vi "thcd_400_main.vi"(3 "variable_ref":T1) -> ()   [LabVIEW 2019]
uses:
  thcd_controls/ctrl_chn_thcd.ctl
  thcd_controls/variable_reference.ctl
  thcd_controls/ctrl_sms_thcd.ctl
  thcd_commands/thcd_set_samp.vi
panel:
  out "thcd_st_ch2":bool caption="Status"
  out "thcd_res_msg_ch2":string caption="Msg"
  in  "thcd_val_ch2":dbl caption="SP (V)" min=0.0 max=100.0 step=1.0 format="%#.6g"
  in  "set_ch2":bool
  out "Last Updated":timestamp format="%<%Y-%m-%d %H:%M:%S>T"
  out "Sensor data":cluster{cluster{"X":dbl, "Y":dbl}[]}[](graph)
  out "thcd_st":bool caption="Status"
  out "thcd_res_msg":string caption="Msg"
  in  "thcd_val":dbl caption="SP (V)" min=0.0 max=100.0 step=1.0 format="%#.6g"
  in  "milliseconds to wait":u32=1000
  out "thcd_res_4":T3
  out "thcd_res_3":T3
  out "thcd_res_2":T3
  out "thcd_res_1":T3
  in  "getstat":bool
  in  "set":bool
  in  "read":bool
  out "res_ch3":dbl
  out "res_ch2":dbl
  out "res_ch1":dbl
  in  "Baud_rate":u32(ring)=9600 items=["9.6KHz"=9600, "19.2KHz"=19200]
  in  "thcd_visa":refnum<visa-resource-name>="COM13"
  in  "Init Devices":bool
  in  "Exit":bool
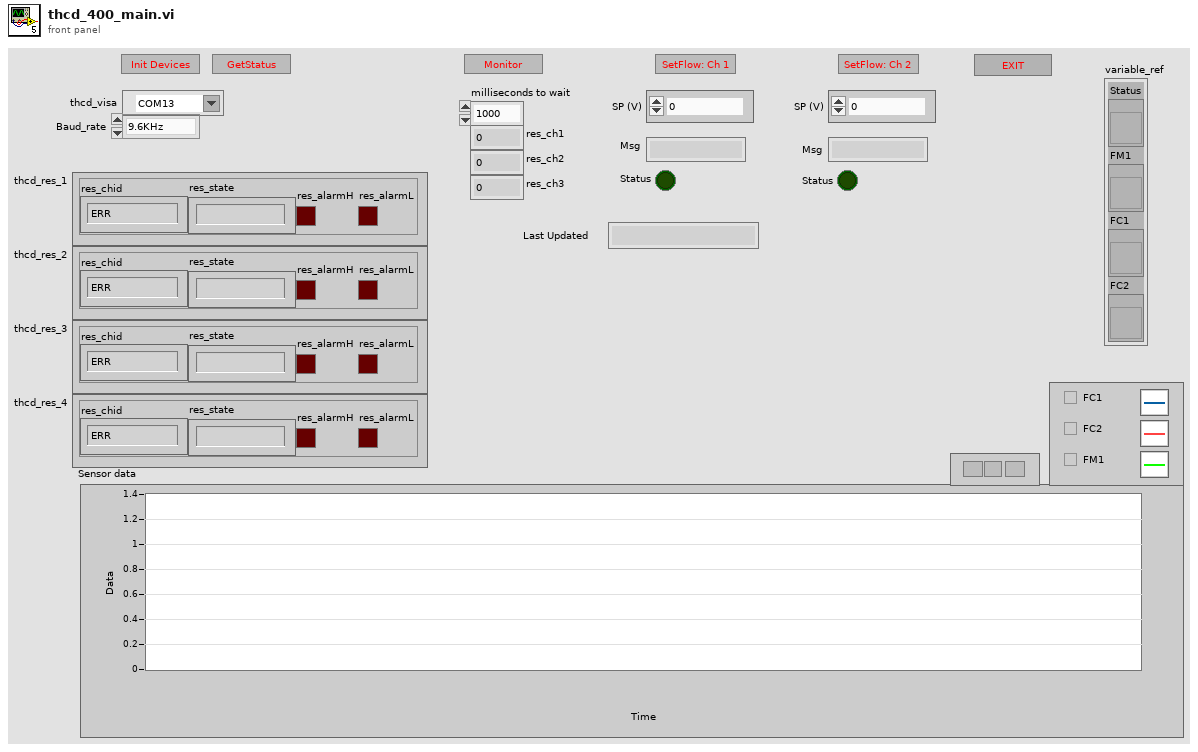
[diagram p1: front panel]
types:
  T1 = typedef "variable_reference.ctl" = cluster{"Status":refnum<vi>, "FM1":refnum<vi>, "FC1":refnum<vi>, "FC2":refnum<vi>}
  T2 = typedef "ctrl_chn_thcd.ctl" = enum8{"ERR", "1", "2", "3", "4"}
  T3 = cluster{"res_chid":T2, "res_state":string, "res_alarmH":bool, "res_alarmL":bool}
  T4 = typedef "ctrl_sms_thcd.ctl" = enum16{"idle", "init", "exit", "read", "set", "set_ch2", "getstat"}
  T5 = enum16{"SetPoint", "AlarmH", "AlarmL", "Multiplier", "CalibValue"}
  T6 = cluster{"res_chid":T2, "res_val":dbl, "res_uom":string, "res_gid":string}[]
  T7 = cluster{"res_chid":T2, "res_val":dbl, "res_uom":string, "res_gid":string}
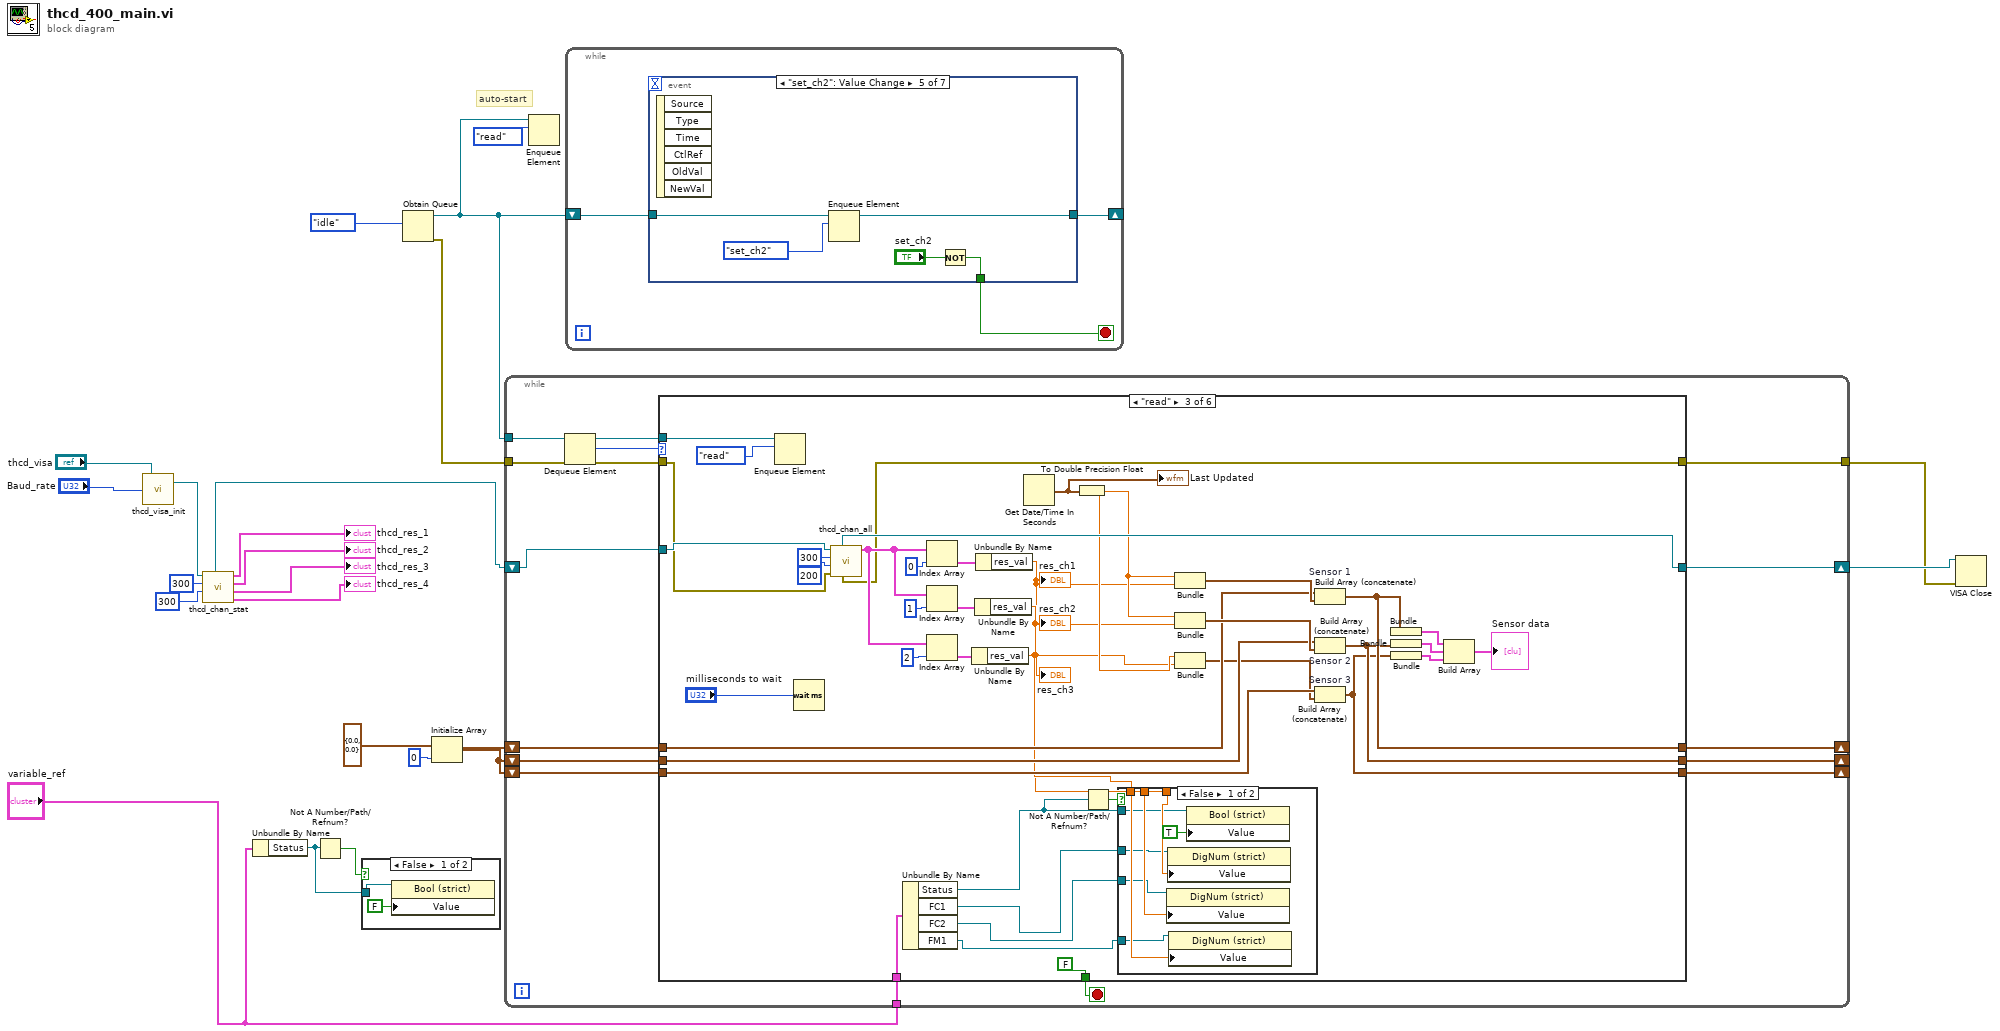
[diagram p0: block diagram]
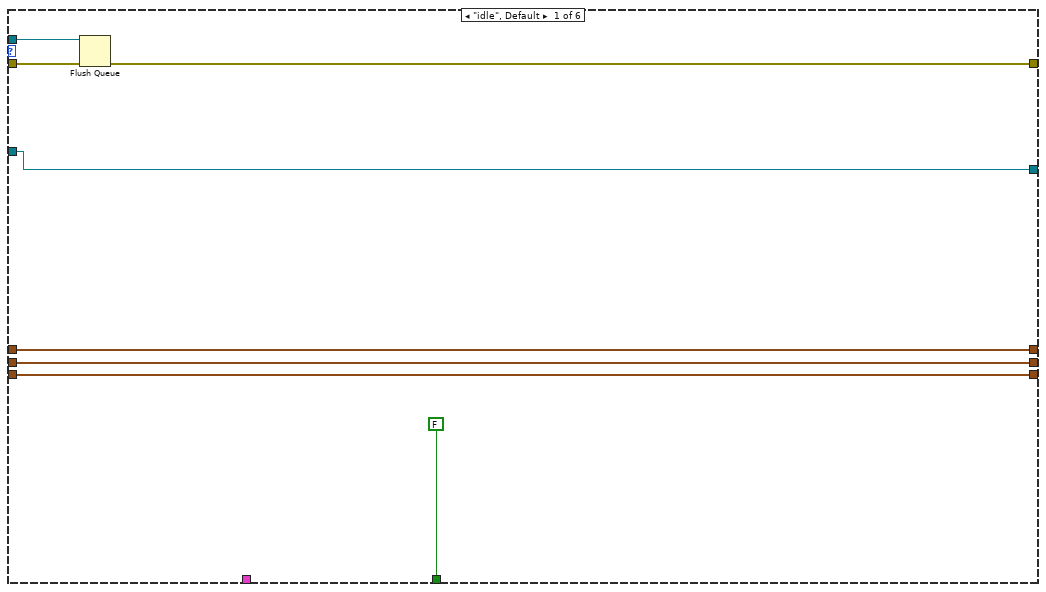
[diagram p3: hidden frame]
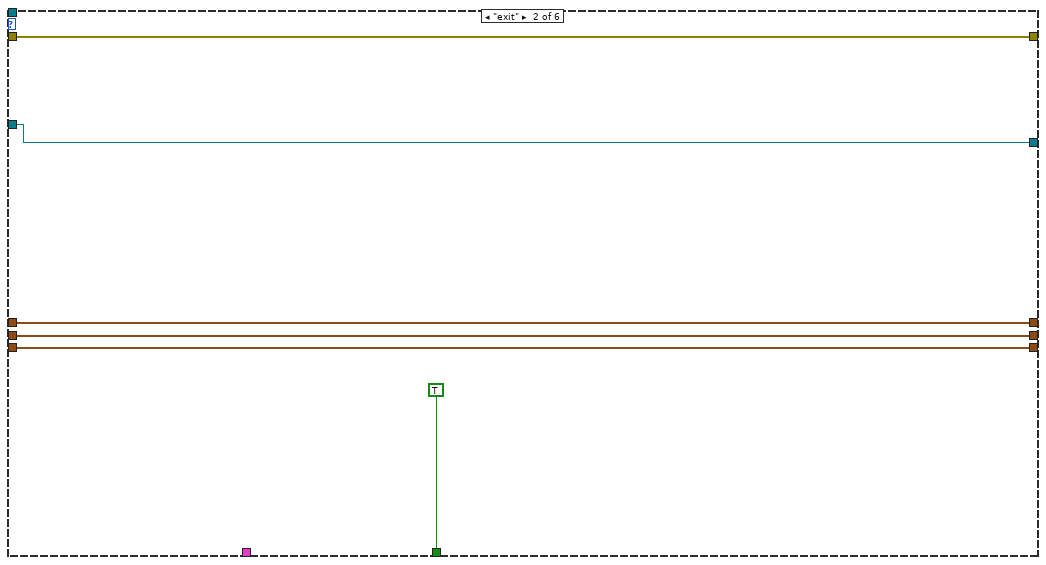
[diagram p4: hidden frame]
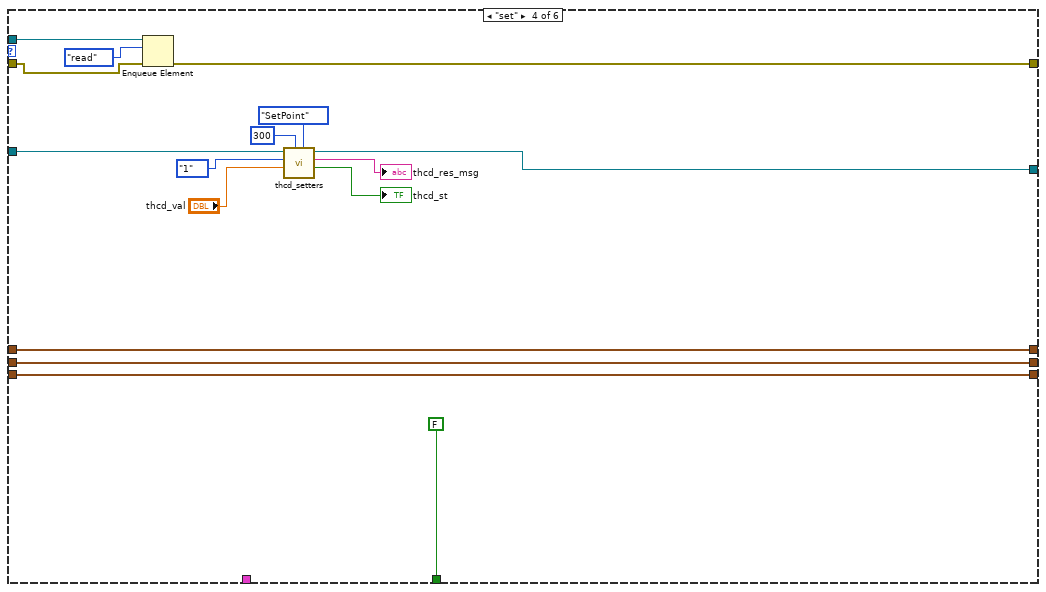
[diagram p6: hidden frame]
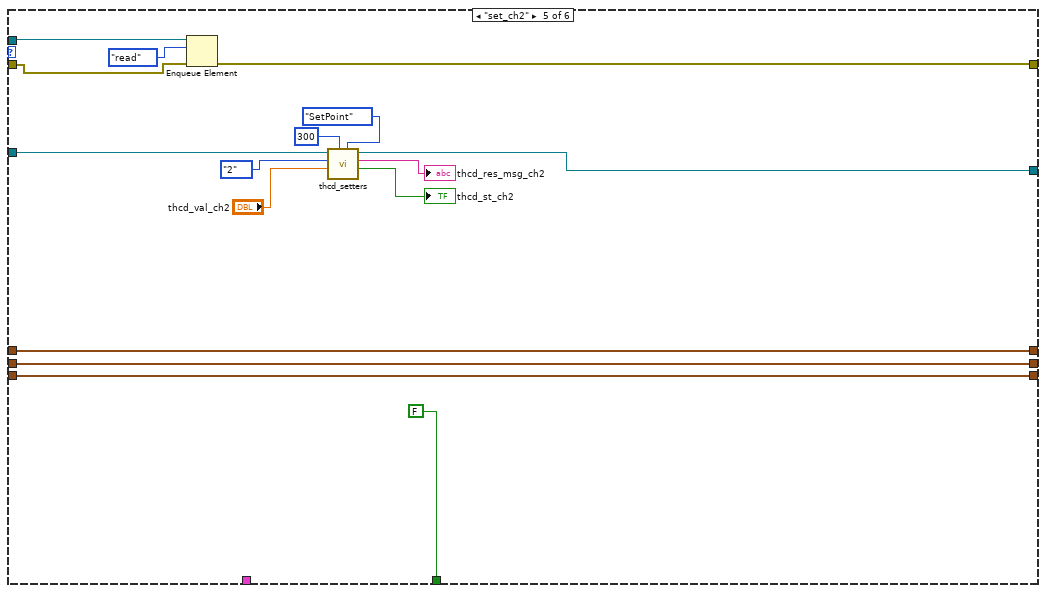
[diagram p7: hidden frame]
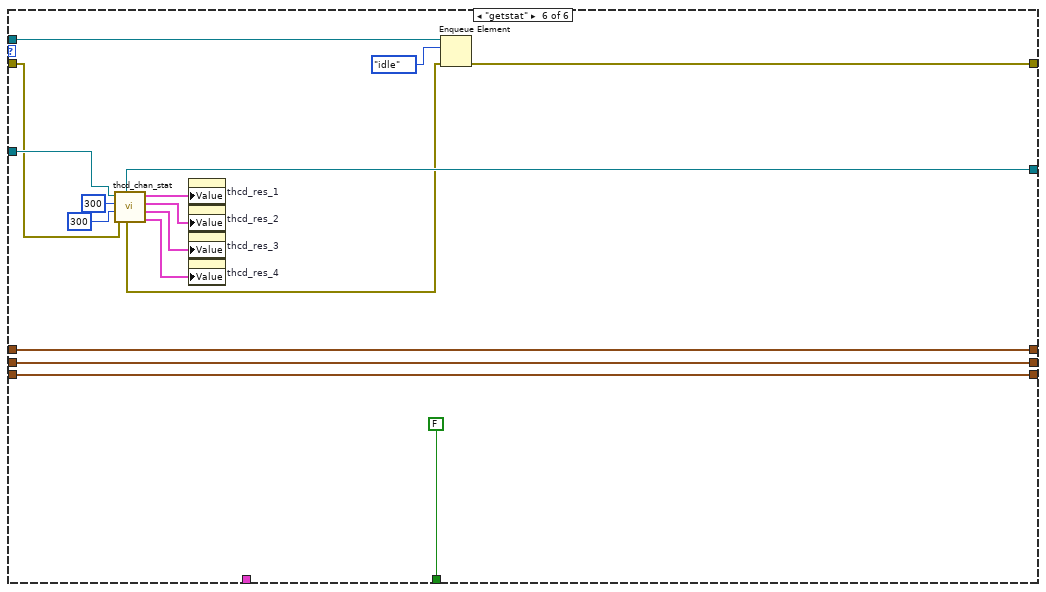
[diagram p8: hidden frame]
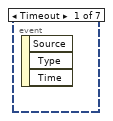
[diagram p9: hidden frame]
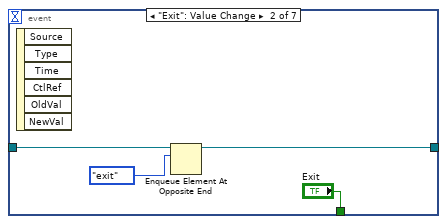
[diagram p10: hidden frame]
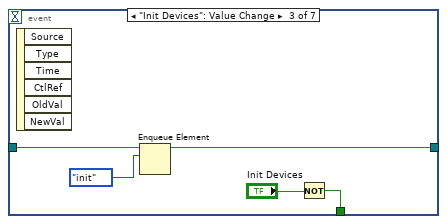
[diagram p11: hidden frame]
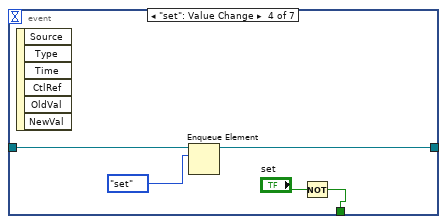
[diagram p12: hidden frame]
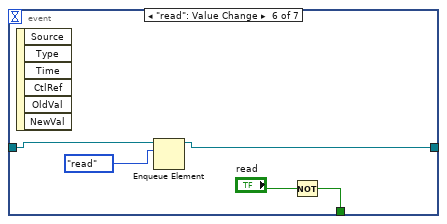
[diagram p13: hidden frame]
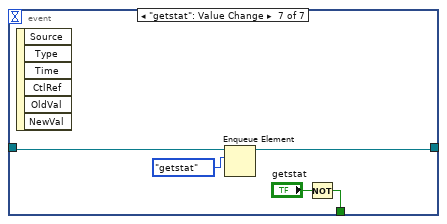
[diagram p14: hidden frame]
diagram:
  # "auto-start"
  n1 = call "thcd_visa_init.vi"("Serial Settings:Baud Rate"="Baud_rate", "thcd_visa"="thcd_visa") -> ("thcd_visa"=w9:refnum<visa-resource-name>)  [unwired: 1 in, 1 out]
  n2 = call "thcd_chan_stat.vi"("thcd_b2r"=u32 300, "thcd_delay"=u32 300, "thcd_visa"=w9) -> ("thcd_res_4"=→"thcd_res_4":T3, "thcd_res_3"=→"thcd_res_3":T3, "thcd_res_2"=→"thcd_res_2":T3, "thcd_res_1"=→"thcd_res_1":T3, "thcd_visa"=w8:refnum<visa-resource-name>)  [unwired: 1 in, 3 out]
  n3 = Unbundle By Name("variable_ref") -> ("Status"=w2:refnum<vi>)
  n4 = Not A Number/Path/Refnum?(number/path/refnum=w2) -> (NaN/Path/Refnum?=w1:bool)
  n5 = case shown="False" w1 {
    tunnel: w2 -> [w24 _]
    frame False {
      n6 = property class="Bool (strict)"(reference=w24, "Value"=FALSE) -> ()  [unwired: 1 in, 2 out]
    }
    frame True {
    }
  }
  n7 = Obtain Queue(element data type=ctrl_sms_thcd."idle" ("Enum")) -> (queue out=w6:refnum<queue>, error out=w21:errorcluster)  [unwired: 4 in, 1 out]
  n8 = Initialize Array(cluster{"X":dbl, "Y":dbl} {"X"=0.0, "Y"=0.0}, 0 ("dimension size")) -> (w18:cluster{"X":dbl, "Y":dbl}[])
  n9 = while {
    tunnel: w21 -> [w38]
    tunnel: [w35] -> w3
    tunnel: w6 -> [w39]
    shift-right: [w26] -> w4
    shift-left: w8 -> [w33]
    shift-right: [w29] -> _
    shift-left: w18 -> [w32]
    shift-right: [w28] -> _
    shift-left: w18 -> [w31]
    shift-right: [w27] -> _
    shift-left: w18 -> [w30]
    tunnel: "variable_ref" -> [w25]
    stop <- w40 stop-if-true
    n10 = Dequeue Element(queue=w39, error in (no error)=w38) -> (queue out=w34:refnum<queue>, element=w37:T4, error out=w36:errorcluster)  [unwired: 1 in, 1 out]
    n11 = case shown="\"read\"" w37 {
      tunnel: w34 -> [w47 _ w79 w117 w128 w151]
      tunnel: [FALSE TRUE FALSE FALSE FALSE FALSE] -> w40
      tunnel: w36 -> [w46 w53 w94 w116 w127 w137]
      tunnel: [w45 w53 w83 w115 w126 w150] -> w35
      tunnel: [w44 w52 w91 w113 w120 w142] -> w26
      tunnel: w33 -> [w44 w52 w95 w114 w125 w143]
      tunnel: w32 -> [w43 w51 w72 w106 w123 w148]
      tunnel: w31 -> [w42 w50 w71 w105 w122 w147]
      tunnel: w30 -> [w41 w49 w70 w104 w121 w146]
      tunnel: [w43 w51 w67 w106 w123 w148] -> w29
      tunnel: [w42 w50 w66 w105 w122 w147] -> w28
      tunnel: [w41 w49 w65 w104 w121 w146] -> w27
      tunnel: w25 -> [_ _ w59 _ _ _]
      frame "idle", Default {
        n12 = Flush Queue(queue=w47, error in (no error)=w46) -> (error out=w45:errorcluster)  [unwired: 2 out]
      }
      frame "exit" {
      }
      frame "read" {
        n13 = Enqueue Element(queue=w79, element=ctrl_sms_thcd."read") -> ()  [unwired: 2 in, 3 out]
        n14 = Wait (ms)(milliseconds to wait="milliseconds to wait") -> ()  [unwired: 1 out]
        n15 = call "thcd_chan_all.vi"("err_in"=w94, "thcd_b2r"=u32 200, "thcd_delay"=u32 300, "thcd_visa"=w95) -> ("thcd_res"=w84:T6, "err_out"=w83:errorcluster, "thcd_visa"=w91:refnum<visa-resource-name>)  [unwired: 3 in, 2 out]
        n16 = Unbundle By Name(w59) -> ("Status"=w60:refnum<vi>, "FC1"=w61:refnum<vi>, "FC2"=w62:refnum<vi>, "FM1"=w63:refnum<vi>)
        n17 = Index Array(array=w84, index=0) -> (element=w89:T7)
        n18 = Index Array(array=w84, index=1) -> (element=w88:T7)
        n19 = Index Array(array=w84, index=2) -> (element=w87:T7)
        n20 = Unbundle By Name(w87) -> ("res_val"=w58:dbl)
        "res_ch3" <- w58
        n21 = Unbundle By Name(w88) -> ("res_val"=w57:dbl)
        "res_ch2" <- w57
        n22 = Unbundle By Name(w89) -> ("res_val"=w56:dbl)
        "res_ch1" <- w56
        n23 = Get Date/Time In Seconds() -> (seconds since 1Jan1904=w55:timestamp)
        "Last Updated" <- w55
        n24 = To Double Precision Float(number=w55) -> (double precision float=w73:dbl)
        n25 = Not A Number/Path/Refnum?(number/path/refnum=w60) -> (NaN/Path/Refnum?=w64:bool)
        n26 = case shown="False" w64 {
          tunnel: w56 -> [w103 _]
          tunnel: w57 -> [w102 _]
          tunnel: w58 -> [w101 _]
          tunnel: w61 -> [w100 _]
          tunnel: w62 -> [w99 _]
          tunnel: w63 -> [w98 _]
          tunnel: w60 -> [w97 _]
          frame False {
            n27 = property class="DigNum (strict)"(reference=w99, "Value"=w102) -> ()  [unwired: 1 in, 2 out]
            n28 = property class="DigNum (strict)"(reference=w100, "Value"=w103) -> ()  [unwired: 1 in, 2 out]
            n29 = property class="DigNum (strict)"(reference=w98, "Value"=w101) -> ()  [unwired: 1 in, 2 out]
            n30 = property class="Bool (strict)"(reference=w97, "Value"=TRUE) -> ()  [unwired: 1 in, 2 out]
          }
          frame True {
          }
        }
        n31 = Bundle(w73, "res_val"=w56) -> (w78:cluster{dbl, "res_val":dbl})  [unwired: 1 in]
        n32 = Bundle(w73, "res_val"=w57) -> (w74:cluster{dbl, "res_val":dbl})  [unwired: 1 in]
        n33 = Bundle(w73, "res_val"=w58) -> (w69:cluster{dbl, "res_val":dbl})  [unwired: 1 in]
        n34 = Build Array (concatenate) "Sensor 1"(w72, w78) -> (w67:cluster{"X":dbl, "res_val":dbl}[])
        n35 = Build Array (concatenate) "Sensor 2"(w71, w74) -> (w66:cluster{"X":dbl, "res_val":dbl}[])
        n36 = Build Array (concatenate) "Sensor 3"(w70, w69) -> (w65:cluster{"X":dbl, "res_val":dbl}[])
        n37 = Bundle(w67) -> (w77:cluster{cluster{"X":dbl, "res_val":dbl}[]})  [unwired: 1 in]
        n38 = Bundle(w66) -> (w75:cluster{cluster{"X":dbl, "res_val":dbl}[]})  [unwired: 1 in]
        n39 = Bundle(w65) -> (w68:cluster{cluster{"X":dbl, "res_val":dbl}[]})  [unwired: 1 in]
        n40 = Build Array(w77, w75, w68) -> (→"Sensor data":cluster{cluster{"X":dbl, "res_val":dbl}[]}[])
      }
      frame "set" {
        n41 = Enqueue Element(queue=w117, element=ctrl_sms_thcd."read", error in (no error)=w116) -> (error out=w115:errorcluster)  [unwired: 1 in, 2 out]
        n42 = call-poly "thcd_setters.vi"("thcd_com"=T5."SetPoint", "thcd_delay"=u32 300, "thcd_val"="thcd_val", "thcd_ch"=ctrl_chn_thcd."1", "thcd_visa"=w114) -> ("thcd_st"=→"thcd_st":bool, "thcd_res_msg"=→"thcd_res_msg":string, "thcd_visa"=w113:refnum<visa-resource-name>)  [unwired: 1 in, 1 out]
      }
      frame "set_ch2" {
        n43 = Enqueue Element(queue=w128, element=ctrl_sms_thcd."read", error in (no error)=w127) -> (error out=w126:errorcluster)  [unwired: 1 in, 2 out]
        n44 = call-poly "thcd_setters.vi"("thcd_com"=T5."SetPoint", "thcd_delay"=u32 300, "thcd_val"="thcd_val_ch2", "thcd_ch"=ctrl_chn_thcd."2", "thcd_visa"=w125) -> ("thcd_st"=→"thcd_st_ch2":bool, "thcd_res_msg"=→"thcd_res_msg_ch2":string, "thcd_visa"=w120:refnum<visa-resource-name>)  [unwired: 1 in, 1 out]
      }
      frame "getstat" {
        n45 = call "thcd_chan_stat.vi"("err_in"=w137, "thcd_b2r"=u32 300, "thcd_delay"=u32 300, "thcd_visa"=w143) -> ("thcd_res_4"=w138:T3, "thcd_res_3"=w139:T3, "thcd_res_2"=w140:T3, "thcd_res_1"=w141:T3, "err_out"=w136:errorcluster, "thcd_visa"=w142:refnum<visa-resource-name>)  [unwired: 2 out]
        n46 = property on="thcd_res_1" class="Clust (strict)"("Value"=w141) -> ()  [unwired: 2 in, 2 out]
        n47 = property on="thcd_res_2" class="Clust (strict)"("Value"=w140) -> ()  [unwired: 2 in, 2 out]
        n48 = property on="thcd_res_3" class="Clust (strict)"("Value"=w139) -> ()  [unwired: 2 in, 2 out]
        n49 = property on="thcd_res_4" class="Clust (strict)"("Value"=w138) -> ()  [unwired: 2 in, 2 out]
        n50 = Enqueue Element(queue=w151, element=ctrl_sms_thcd."idle", error in (no error)=w136) -> (error out=w150:errorcluster)  [unwired: 1 in, 2 out]
      }
    }
  }
  n51 = Enqueue Element(queue=w6, element=ctrl_sms_thcd."read") -> ()  [unwired: 2 in, 3 out]
  n52 = while {
    shift-right: [w154] -> _
    shift-left: w6 -> [w155]
    stop <- w153 stop-if-true
    n53 = event shown="[4] \"set_ch2\": Value Change" {
      selector: _ -> [_ _ _ _ _ _ _]
      dyn-events: _ -> [_ _ _ _ _ _ _]
      timeout: _ -> [_ _ _ _ _ _ _]
      tunnel: w155 -> [_ w159 w164 w166 w171 w177 w182]
      tunnel: [_ w158 w163 w165 w170 w176 w181] -> w154
      tunnel: [_ "Exit" w160 w168 w173 w178 w183] -> w153
      event Timeout {
        n54 = event-data() -> ()  [unwired: 1 in, 3 out]
      }
      event "Exit": Value Change {
        n55 = event-data() -> ()  [unwired: 1 in, 6 out]
        n56 = Enqueue Element At Opposite End(queue=w159, element=ctrl_sms_thcd."exit" ("Enum")) -> (queue out=w158:refnum<queue>)  [unwired: 2 in, 2 out]
      }
      event "Init Devices": Value Change {
        n57 = event-data() -> ()  [unwired: 1 in, 6 out]
        n58 = Enqueue Element(queue=w164, element=ctrl_sms_thcd."init") -> (queue out=w163:refnum<queue>)  [unwired: 2 in, 2 out]
        n59 = Not(x="Init Devices") -> (.not. x?=w160:bool)
      }
      event "set": Value Change {
        n60 = event-data() -> ()  [unwired: 1 in, 6 out]
        n61 = Enqueue Element(queue=w166, element=ctrl_sms_thcd."set" ("Enum")) -> (queue out=w165:refnum<queue>)  [unwired: 2 in, 2 out]
        n62 = Not(x="set") -> (.not. x?=w168:bool)
      }
      event "set_ch2": Value Change {
        n63 = event-data() -> ()  [unwired: 1 in, 6 out]
        n64 = Enqueue Element(queue=w171, element=ctrl_sms_thcd."set_ch2" ("Enum")) -> (queue out=w170:refnum<queue>)  [unwired: 2 in, 2 out]
        n65 = Not(x="set_ch2") -> (.not. x?=w173:bool)
      }
      event "read": Value Change {
        n66 = event-data() -> ()  [unwired: 1 in, 6 out]
        n67 = Enqueue Element(queue=w177, element=ctrl_sms_thcd."read" ("Enum")) -> (queue out=w176:refnum<queue>)  [unwired: 2 in, 2 out]
        n68 = Not(x="read") -> (.not. x?=w178:bool)
      }
      event "getstat": Value Change {
        n69 = event-data() -> ()  [unwired: 1 in, 6 out]
        n70 = Enqueue Element(queue=w182, element=ctrl_sms_thcd."getstat") -> (queue out=w181:refnum<queue>)  [unwired: 2 in, 2 out]
        n71 = Not(x="getstat") -> (.not. x?=w183:bool)
      }
    }
  }
  n72 = VISA Close(VISA resource name=w4, error in (no error)=w3) -> ()  [unwired: 1 out]
